vi "Main.vi"() -> ()   [LabVIEW 2012]
uses:
  Consumer Message.ctl
panel:
  out "消费者关闭？":bool
  out "待执行状态":string
  out "高优先级？":bool
  out "积压空间":u8(slide) scale=0.0..100.0
  out "已处理值":i32
  in  "高优先级消息":bool
  in  "标准优先级消息":bool
  in  "停止":bool
  # "待入队处理的消息数量"
  # "消费者循环中当前正在处理的数据"
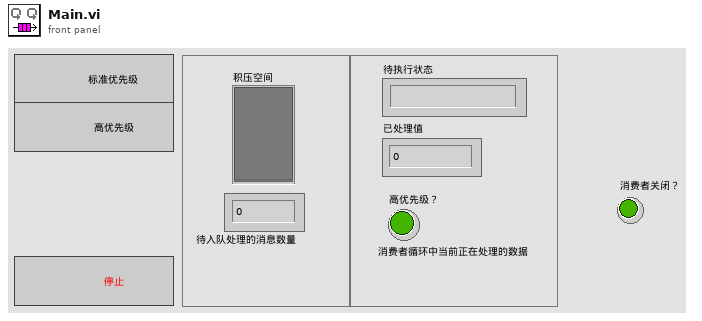
[diagram p1: front panel]
types:
  T1 = typedef "Consumer Message.ctl" = cluster{"消费者状态":string, "布尔数据":bool, "数值数据":i32, "错误":cluster{"状态":bool, "代码":i32, "源":string}}
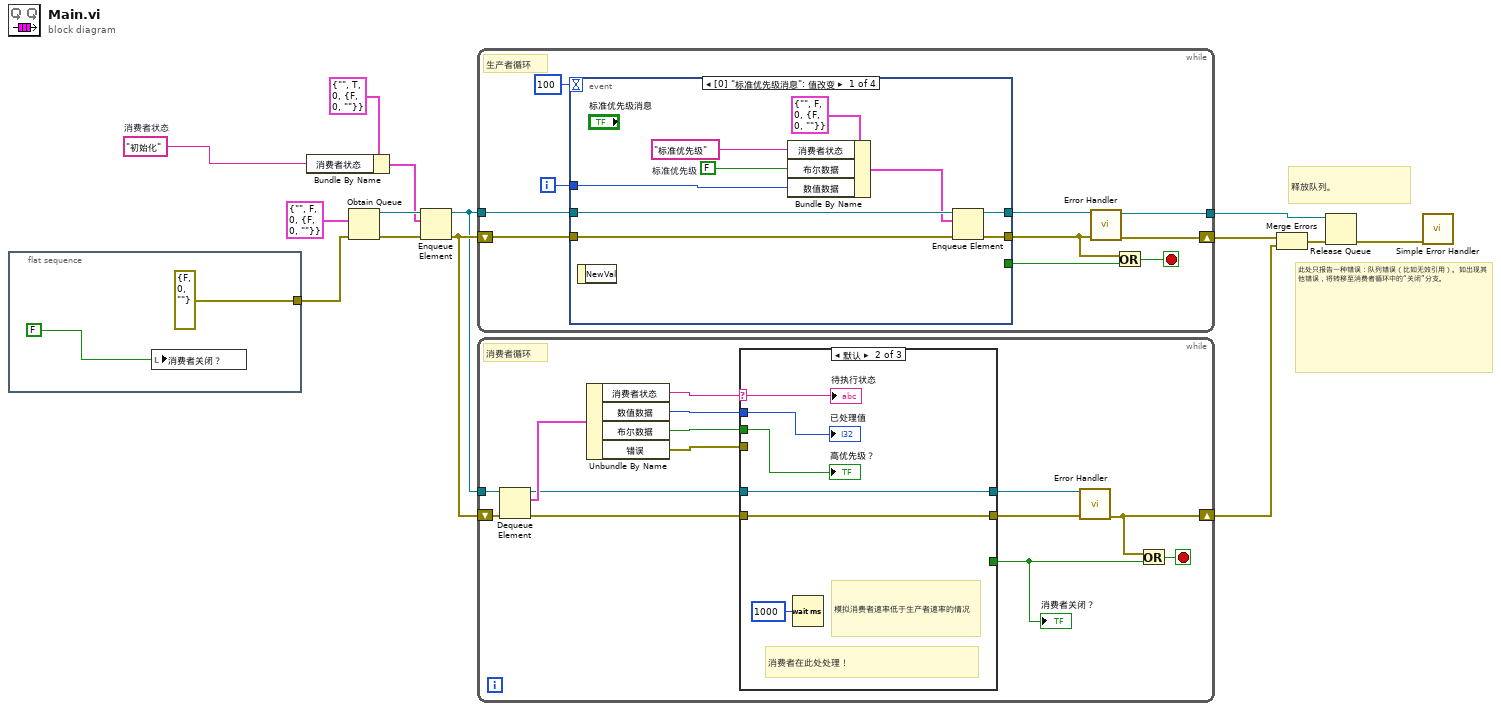
[diagram p0: block diagram]
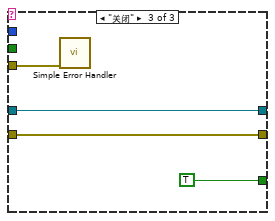
[diagram p3: hidden frame]
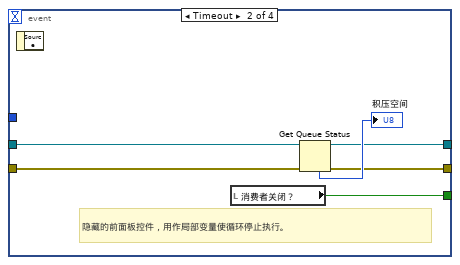
[diagram p4: hidden frame]
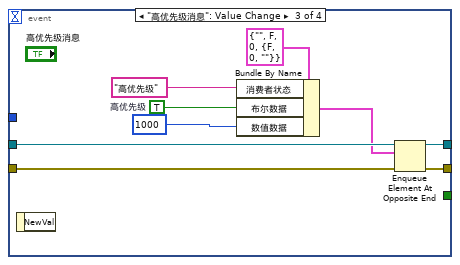
[diagram p5: hidden frame]
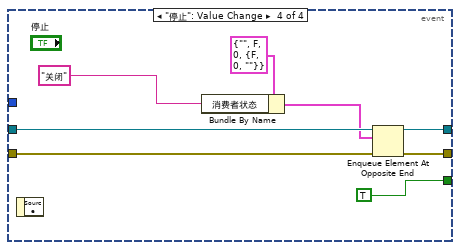
[diagram p6: hidden frame]
diagram:
  w6 = "初始化"  # 消费者状态
  # "释放队列。"
  # "此处只报告一种错误：队列错误（比如无效引用）。如出现其他错误，将转移至消费者循环中的“关闭”分支。"
  n1 = flat-sequence {
    tunnel: [cluster{"状态":bool, "代码":i32, "源":string} {"状态"=FALSE, "代码"=0, "源"=""} ("错误输入（无错误）")] -> w9
    frame #0 {
      n2 = local write "消费者关闭？"(FALSE ("停止循环（局部）")) -> ()
    }
  }
  n3 = Bundle By Name ("按名称捆绑")(cluster=T1 {"消费者状态"="", "布尔数据"=TRUE, "数值数据"=0, "错误"={"状态"=FALSE, "代码"=0, "源"=""}} ("消费者消息"), "消费者状态"=w6) -> (w7:T1)
  n4 = Obtain Queue ("获取队列引用")(element data type=T1 {"消费者状态"="", "布尔数据"=FALSE, "数值数据"=0, "错误"={"状态"=FALSE, "代码"=0, "源"=""}}, error in (no error)=w9) -> (queue out=w11:refnum<queue>, error out=w14:errorcluster)  [unwired: 3 in, 1 out]
  n5 = Enqueue Element ("元素入队列")(queue=w11, element=w7, error in (no error)=w14) -> (queue out=w10:refnum<queue>, error out=w12:errorcluster)  [unwired: 1 in, 1 out]
  n6 = while {
    tunnel: w10 -> [w26]
    shift-right: [w18] -> w5
    shift-left: w12 -> [w25]
    tunnel: [w17] -> w1
    i -> [w24]
    stop <- w20 stop-if-true
    # "生产者循环"
    n7 = event shown="[0] \"标准优先级消息\": 值改变" {
      selector: _ -> [_ _ _ _]
      dyn-events: _ -> [_ _ _ _]
      timeout: 100 -> [_ _ _ _]
      tunnel: w26 -> [w35 w39 w49 w58]
      tunnel: w25 -> [w33 w38 w48 w56]
      tunnel: [w34 w37 w50 w55] -> w19
      tunnel: [_ w41 _ TRUE] -> w21
      tunnel: w24 -> [w32 _ _ _]
      tunnel: [w28 w36 w44 w54] -> w23
      event "标准优先级消息": Value Change {
        w29 = FALSE  # 标准优先级
        n8 = event-data ("事件数据节点")() -> ()  [unwired: 1 in, 1 out]
        n9 = Bundle By Name ("按名称捆绑")(cluster=T1 {"消费者状态"="", "布尔数据"=FALSE, "数值数据"=0, "错误"={"状态"=FALSE, "代码"=0, "源"=""}}, "消费者状态"="标准优先级" ("字符串数据"), "布尔数据"=w29, "数值数据"=w32) -> (w31:T1)
        n10 = Enqueue Element ("元素入队列")(queue=w35, element=w31, error in (no error)=w33) -> (queue out=w28:refnum<queue>, error out=w34:errorcluster)  [unwired: 1 in, 1 out]
      }
      event Timeout {
        # "隐藏的前面板控件，用作局部变量使循环停止执行。"
        n11 = event-data ("事件数据节点")() -> ()  [unwired: 1 in, 1 out]
        n12 = local read "消费者关闭？"() -> (w41:bool)
        n13 = Get Queue Status ("获取队列状态")(queue=w39, error in (no error)=w38) -> (queue out=w36:refnum<queue>, error out=w37:errorcluster, # elements in queue=→"积压空间":i32)  [unwired: 1 in, 5 out]
      }
      event "高优先级消息": Value Change {
        w43 = TRUE  # 高优先级
        n14 = event-data ("事件数据节点")() -> ()  [unwired: 1 in, 1 out]
        n15 = Bundle By Name ("按名称捆绑")(cluster=T1 {"消费者状态"="", "布尔数据"=FALSE, "数值数据"=0, "错误"={"状态"=FALSE, "代码"=0, "源"=""}}, "消费者状态"="高优先级" ("字符串数据"), "布尔数据"=w43, "数值数据"=1000) -> (w46:T1)
        n16 = Enqueue Element At Opposite End ("队列最前端插入元素")(queue=w49, element=w46, error in (no error)=w48) -> (queue out=w44:refnum<queue>, error out=w50:errorcluster)  [unwired: 1 in, 1 out]
      }
      event "停止": Value Change {
        n17 = event-data ("事件数据节点")() -> ()  [unwired: 1 in, 1 out]
        n18 = Bundle By Name ("按名称捆绑")(cluster=T1 {"消费者状态"="", "布尔数据"=FALSE, "数值数据"=0, "错误"={"状态"=FALSE, "代码"=0, "源"=""}}, "消费者状态"="关闭") -> (w51:T1)
        n19 = Enqueue Element At Opposite End ("队列最前端插入元素")(queue=w58, element=w51, error in (no error)=w56) -> (queue out=w54:refnum<queue>, error out=w55:errorcluster)  [unwired: 1 in, 1 out]
      }
    }
    n20 = call "Error Handler.vi"("错误输入"=w19, "队列输入"=w23) -> ("错误输出"=w18:cluster{"状态":bool, "代码":i32, "源":string}, "队列输出"=w17:refnum<queue>)  [unwired: 8 in]
    n21 = Or ("或")(x=w19, y=w21) -> (x .or. y?=w20:bool)
  }
  n22 = while {
    tunnel: w10 -> [w72]
    shift-right: [w61] -> w4
    shift-left: w12 -> [w71]
    stop <- w62 stop-if-true
    # "消费者循环"
    n23 = Dequeue Element ("元素出队列")(queue=w72, error in (no error)=w71) -> (queue out=w60:refnum<queue>, element=w70:T1, error out=w59:errorcluster)  [unwired: 1 in, 1 out]
    n24 = Unbundle By Name ("按名称解除捆绑")(w70) -> ("消费者状态"=w69:string, "数值数据"=w68:i32, "布尔数据"=w67:bool, "错误"=w64:cluster{"状态":bool, "代码":i32, "源":string})
    n25 = case shown="默认" w69 {
      selector: w69 -> [_ w77 _]
      tunnel: [_ _ TRUE] -> w63
      tunnel: w59 -> [w73 w75 w81]
      tunnel: [w73 w75 w81] -> w66
      tunnel: w68 -> [_ w80 _]
      tunnel: w67 -> [_ w79 _]
      tunnel: w60 -> [w74 w78 w82]
      tunnel: [w74 w78 w82] -> w65
      tunnel: w64 -> [_ _ w83]
      frame "初始化" {
      }
      frame Default {
        # "模拟消费者速率低于生产者速率的情况"
        # "消费者在此处处理！"
        n26 = Wait (ms) ("等待(ms)")(milliseconds to wait=u32 1000 ("等待时间（毫秒）")) -> ()  [unwired: 1 out]
        "已处理值" <- w80
        "高优先级？" <- w79
        "待执行状态" <- w77
      }
      frame "关闭" {
        n27 = call <vilib>:"Simple Error Handler.vi"("error in (no error)"=w83) -> ()  [unwired: 4 in, 5 out]
      }
    }
    "消费者关闭？" <- w63
    n28 = call "Error Handler.vi"("错误输入"=w66, "队列输入"=w65) -> ("错误输出"=w61:cluster{"状态":bool, "代码":i32, "源":string})  [unwired: 8 in, 1 out]
    n29 = Or ("或")(x=w61, y=w63) -> (x .or. y?=w62:bool)
  }
  n30 = Merge Errors ("合并错误")(w5, w4) -> (w3:errorcluster)
  n31 = Release Queue ("释放队列引用")(queue=w1, error in (no error)=w3) -> (error out=w2:errorcluster)  [unwired: 1 in, 2 out]
  n32 = call <vilib>:"Simple Error Handler.vi"("error in (no error)"=w2) -> ()  [unwired: 4 in, 5 out]
